vi "Define Action.vi"(8 "ErrorIn":errorcluster, 9 "IAction.lvclass":refnum<class "IAction.lvclass">, 10 "Name":string, 11 "TopModuleIn":refnum<class "TopModule.lvclass">) -> (0 "ErrorOut":errorcluster, 3 "TopModuleOut":refnum<class "TopModule.lvclass">)   [LabVIEW 2020, in "TopModule.lvclass"]
uses:
  TopModule.lvclass
  TopModule.lvclass/TopModule.ctl
  IAction/IAction.lvclass
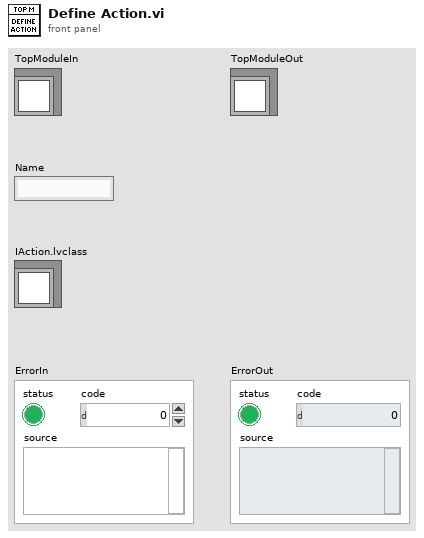
[diagram p1: front panel]
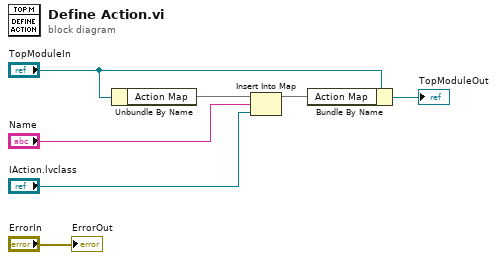
[diagram p0: block diagram]
diagram:
  n1 = Unbundle By Name("TopModuleIn") -> ("Action Map"=w6:map{string, refnum<class "IAction.lvclass">})
  n2 = Insert Into Map(map in=w6, key="Name", value="IAction.lvclass") -> (map out=w2:map{string, refnum<class "IAction.lvclass">})  [unwired: 2 out]
  n3 = Bundle By Name(cluster="TopModuleIn", "Action Map"=w2) -> (→"TopModuleOut":refnum<class "TopModule.lvclass">)
  "ErrorOut" <- "ErrorIn"
